vi "Write to VISA.vi"(8 "error in (no error)":errorcluster, 9 "Right":u8[](array[numeric]), 10 "Left":u8[](array[numeric]), 11 "LED Matrix in":refnum<class "LED Matrix.lvclass">) -> (0 "error out":errorcluster, 3 "LED Matrix out":refnum<class "LED Matrix.lvclass">)   [LabVIEW 2026, in "LED Matrix.lvlib" / "LED Matrix.lvclass"]
uses:
  LED Matrix.lvclass
  LED Matrix.lvclass/LED Matrix.ctl
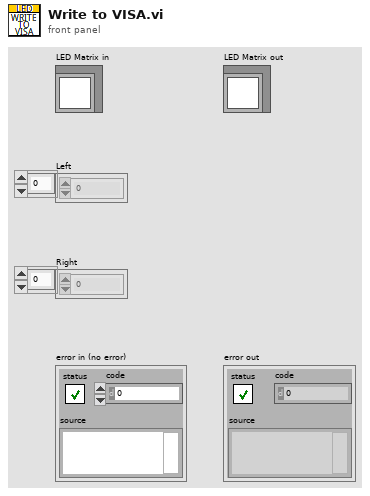
[diagram p1: front panel]
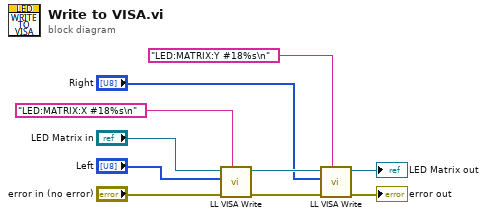
[diagram p0: block diagram]
diagram:
  n1 = call "LL VISA Write.vi"("format string"="LED:MATRIX:X #18%s\n" ("concatenated string"), "error in (no error)"="error in (no error)", "unsigned byte array"="Left", "LED Matrix in"="LED Matrix in") -> ("error out"=w7:errorcluster, "LED Matrix out"=w8:refnum<class "LED Matrix.lvclass">)  [unwired: 6 in]
  n2 = call "LL VISA Write.vi"("format string"="LED:MATRIX:Y #18%s\n" ("concatenated string"), "error in (no error)"=w7, "unsigned byte array"="Right", "LED Matrix in"=w8) -> ("error out"=→"error out":errorcluster, "LED Matrix out"=→"LED Matrix out":refnum<class "LED Matrix.lvclass">)  [unwired: 6 in]
